vi "Check Offset.vi"(7 "source vi name":string, 8 "error in (no error)":errorcluster, 9 "offset":u64 format="%d bytes", 11 "Pointer in":refnum<class "Pointer.lvclass">) -> (0 "error out":errorcluster, 1 "offset":u64 format="%d bytes", 3 "Pointer out":refnum<class "Pointer.lvclass">)   [LabVIEW 2016, in "Memory Manager.lvlib" / "Pointer.lvclass"]
uses:
  Pointer.lvclass
  Out of Bounds.vi
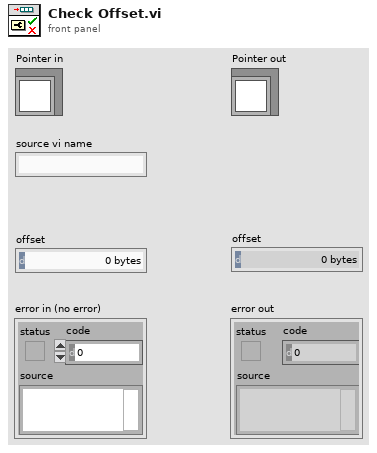
[diagram p1: front panel]
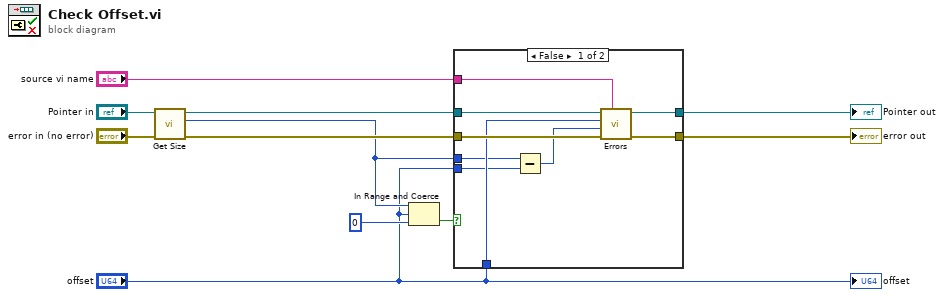
[diagram p0: block diagram]
diagram:
  n1 = call "Get Size.vi"("Pointer in"="Pointer in") -> ("size"=w2:u64, "Pointer out"=w7:refnum<class "Pointer.lvclass">)  [unwired: 9 in]
  n2 = In Range and Coerce(upper limit=w2, x="offset", lower limit=u64 0) -> (In Range?=w8:bool)  [unwired: 1 out]
  n3 = case shown="False" w8 {
    tunnel: w7 -> [w19 w21]
    tunnel: "error in (no error)" -> [w18 w20]
    tunnel: [w17 w21] -> w5
    tunnel: [w16 w20] -> w4
    tunnel: "source vi name" -> [w15 _]
    tunnel: "offset" -> [w14 _]
    tunnel: w2 -> [w13 _]
    tunnel: "offset" -> [w12 _]
    frame False {
      n4 = Subtract(x=w13, y=w12) -> (x-y=w11:u64)
      n5 = call-poly "Errors.vi"("error source vi name"=w15, "error in (no error)"=w18, "size"=w11, "offset"=w14, "Pointer in"=w19) -> ("error out"=w16:errorcluster, "Pointer out"=w17:refnum<class "Pointer.lvclass">)  [unwired: 5 in]
    }
    frame True {
    }
  }
  "error out" <- w4
  "Pointer out" <- w5
  "offset" <- "offset"
